vi "scheduler.vi"(8 "timestampLastFired":dbl, 10 "Hour":i32 min=-23 max=23 step=1, 11 "Day":i32 min=-365 max=7 step=1) -> (0 "timestampNow":dbl, 3 "DoItNow":bool)   [LabVIEW 2022 SP3]
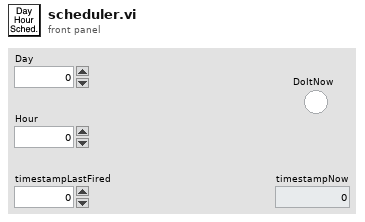
[diagram p1: front panel]
types:
  T1 = typedef "LVDateTimeRec.ctl" = cluster{"fractional second":dbl, "second":i32, "minute":i32, "hour":i32, "day of month":i32, "month":i32, "year":i32, "day of week":i32, "day of year":i32, "DST":i32}
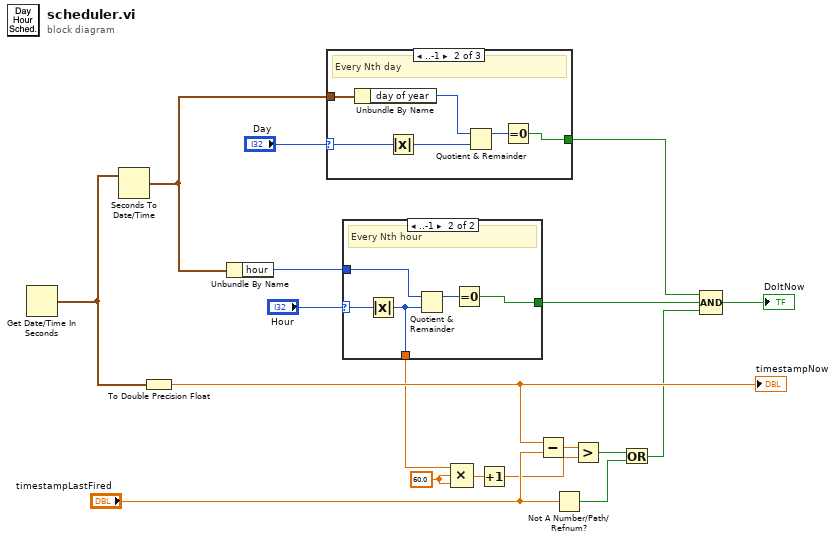
[diagram p0: block diagram]
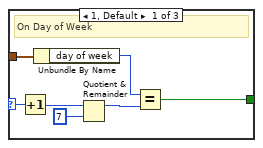
[diagram p2: hidden frame]
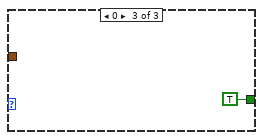
[diagram p3: hidden frame]
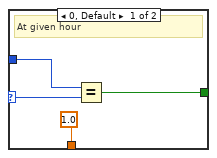
[diagram p4: hidden frame]
diagram:
  w9 = 60.0 ("value")
  n1 = Get Date/Time In Seconds() -> (seconds since 1Jan1904=w12:timestamp)
  n2 = Seconds To Date/Time(time stamp (now)=w12) -> (date time rec=w2:T1)  [unwired: 1 in]
  n3 = To Double Precision Float(number=w12) -> (double precision float=w13:dbl)
  "timestampNow" <- w13
  n4 = Unbundle By Name(w2) -> ("hour"=w7:i32)
  n5 = case shown="..-1" "Day" {
    selector: "Day" -> [w25 w29 _]
    tunnel: [w24 w30 TRUE] -> w1
    tunnel: w2 -> [w23 w27 _]
    frame 1, Default {
      # "On Day of Week"
      n6 = Increment(x=w25) -> (x+1=w21:i32)
      n7 = Unbundle By Name(w23) -> ("day of week"=w22:i32)
      n8 = Quotient & Remainder(x=w21, y=7) -> (x-y*floor(x/y)=w19:i32)  [unwired: 1 out]
      n9 = Equal?(x=w22, y=w19) -> (x = y?=w24:bool)
    }
    frame ..-1 {
      # "Every Nth day"
      n10 = Unbundle By Name(w27) -> ("day of year"=w26:i32)
      n11 = Absolute Value(x=w29) -> (abs(x)=w28:i32)
      n12 = Quotient & Remainder(x=w26, y=w28) -> (x-y*floor(x/y)=w31:i32)  [unwired: 1 out]
      n13 = Equal To 0?(x=w31) -> (x = 0?=w30:bool)
    }
    frame 0 {
    }
  }
  n14 = case shown="..-1" "Hour" {
    selector: "Hour" -> [w35 w39]
    tunnel: [1.0 ("value") w37] -> w8
    tunnel: w7 -> [w34 w38]
    tunnel: [w33 w40] -> w6
    frame 0, Default {
      # "At given hour"
      n15 = Equal?(x=w34, y=w35) -> (x = y?=w33:bool)
    }
    frame ..-1 {
      # "Every Nth hour"
      n16 = Absolute Value(x=w39) -> (abs(x)=w37:i32)
      n17 = Quotient & Remainder(x=w38, y=w37) -> (x-y*floor(x/y)=w41:i32)  [unwired: 1 out]
      n18 = Equal To 0?(x=w41) -> (x = 0?=w40:bool)
    }
  }
  n19 = Compound Arithmetic op=MULTIPLY(w8, w9, w9) -> (w15:dbl)
  n20 = Increment(x=w15) -> (x+1=w10:dbl)
  n21 = Subtract(x=w13, y="timestampLastFired") -> (x-y=w14:dbl)
  n22 = Not A Number/Path/Refnum?(number/path/refnum="timestampLastFired") -> (NaN/Path/Refnum?=w17:bool)
  n23 = Greater?(x=w14, y=w10) -> (0:w16:bool)
  n24 = Or(x=w16, y=w17) -> (x .or. y?=w5:bool)
  n25 = Compound Arithmetic op=AND(w1, w6, w5) -> (→"DoItNow":bool)
